vi "Stack Aligner Tester.vi"(8 "error in (no error)":errorcluster, 10 "Transmitted Light AVI Path":path, 11 "Reflected Light AVI Path":path) -> (0 "error out":errorcluster)   [LabVIEW 2013]
panel:
  out "Offset":cluster{"dx":i32, "dy":i32}
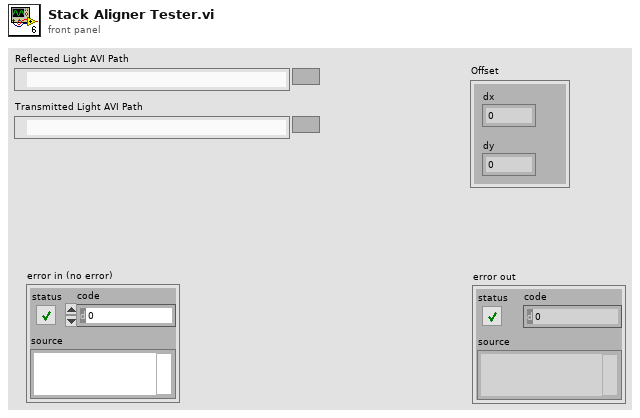
[diagram p1: front panel]
types:
  T1 = typedef "IMAQ Image.ctl" = refnum<image>
  T2 = typedef "Image Type" = u32
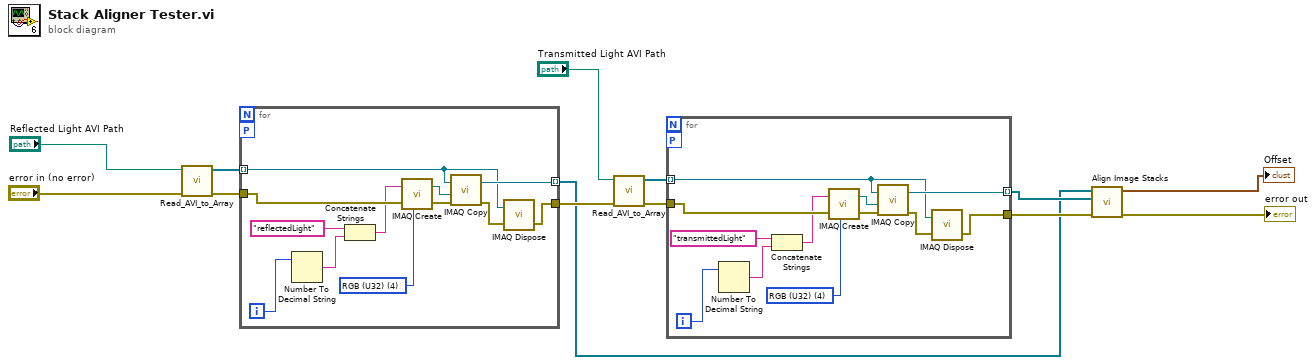
[diagram p0: block diagram]
diagram:
  n1 = call "Read_AVI_to_Array.vi"("Error in (no error)"="error in (no error)", "AVI Path"="Reflected Light AVI Path") -> ("Error out"=w10:errorcluster, "Image Array"=w11:T1[])  [unwired: 7 in, 1 out]
  n2 = for {
    tunnel: w11 -> [w14] mode=indexing
    tunnel: w10 -> [w23]
    tunnel: [w17] -> w3 mode=indexing
    workers-P: _ -> [_]
    tunnel: [w15] -> w6
    i -> [w20]
    w18 = T2 4 items=["Grayscale (U8)", "Grayscale (I16)", "Grayscale (SGL)", "Complex (CSG)", "RGB (U32)", "HSL (U32)", "RGB (U64)", "Grayscale (U16)"] ("Image Type")
    n3 = Number To Decimal String(number=w20) -> (decimal integer string=w21:string)  [unwired: 1 in]
    n4 = Concatenate Strings("reflectedLight", w21) -> (w19:string)
    n5 = call "IMAQ Create"("Image Name"=w19, "Image Type"=w18, "error in (no error)"=w23) -> ("New Image"=w24:T1, "error out"=w25:errorcluster)  [unwired: 2 in]
    n6 = call "IMAQ Copy"("error in (no error)"=w25, "Image Dst"=w24, "Image Src"=w14) -> ("error out"=w16:errorcluster, "Image Dst Out"=w17:T1)  [unwired: 3 in]
    n7 = call "IMAQ Dispose"("Image"=w14, "error in (no error)"=w16) -> ("error out"=w15:errorcluster)  [unwired: 4 in]
  }
  n8 = call "Read_AVI_to_Array.vi"("Error in (no error)"=w6, "AVI Path"="Transmitted Light AVI Path") -> ("Error out"=w9:errorcluster, "Image Array"=w8:T1[])  [unwired: 7 in, 1 out]
  n9 = for {
    tunnel: w8 -> [w27] mode=indexing
    tunnel: w9 -> [w35]
    tunnel: [w29] -> w4 mode=indexing
    workers-P: _ -> [_]
    tunnel: [w26] -> w5
    i -> [w32]
    w30 = T2 4 items=["Grayscale (U8)", "Grayscale (I16)", "Grayscale (SGL)", "Complex (CSG)", "RGB (U32)", "HSL (U32)", "RGB (U64)", "Grayscale (U16)"] ("Image Type")
    n10 = Number To Decimal String(number=w32) -> (decimal integer string=w33:string)  [unwired: 1 in]
    n11 = Concatenate Strings("transmittedLight", w33) -> (w31:string)
    n12 = call "IMAQ Create"("Image Name"=w31, "Image Type"=w30, "error in (no error)"=w35) -> ("New Image"=w36:T1, "error out"=w37:errorcluster)  [unwired: 2 in]
    n13 = call "IMAQ Copy"("error in (no error)"=w37, "Image Dst"=w36, "Image Src"=w27) -> ("error out"=w28:errorcluster, "Image Dst Out"=w29:T1)  [unwired: 3 in]
    n14 = call "IMAQ Dispose"("Image"=w27, "error in (no error)"=w28) -> ("error out"=w26:errorcluster)  [unwired: 4 in]
  }
  n15 = call "Align Image Stacks.vi"("error in (no error)"=w5, "Transmitted Light Stack"=w4, "Reflected Light Stack"=w3) -> ("error out"=→"error out":errorcluster, "Offset"=→"Offset":cluster{"dx":i32, "dy":i32})  [unwired: 7 in]
